vi "Plot V.vi"(7 "Channel number":i32=4, 8 "XY Graph REF":refnum<vi>, 10 "V":bool, 11 "plot setting REF":refnum<vi>) -> ()   [LabVIEW 2023]
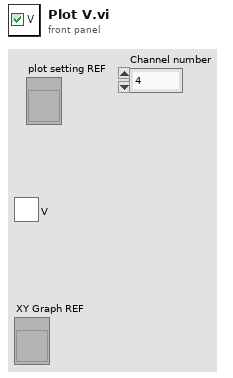
[diagram p1: front panel]
types:
  T1 = cluster{"V plot":bool, "I plot":bool, "Plot colour":u32, "Channel name\n":string}[]
  T2 = cluster{bool, bool, "Plot colour":u32, "Channel name\n":string}
  T3 = cluster{bool, "I plot":bool, "Plot colour":u32, "Channel name\n":string}
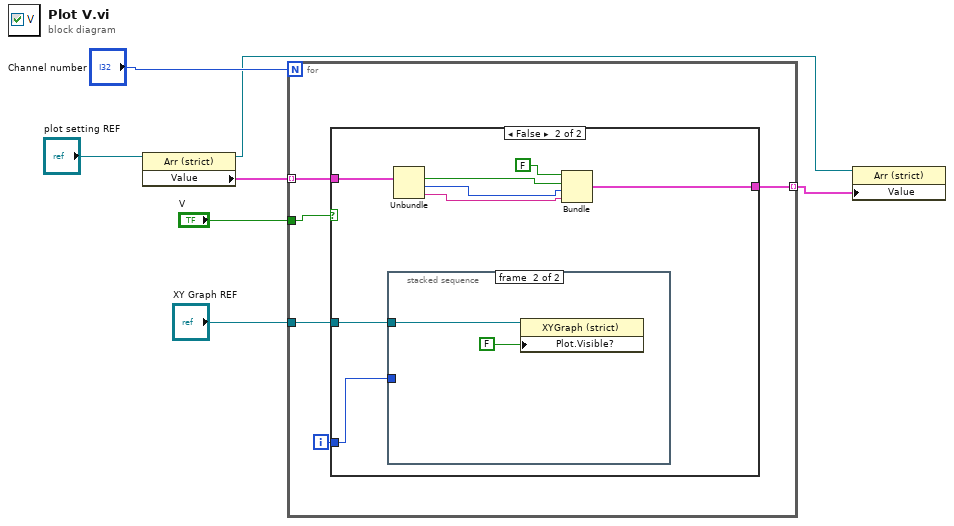
[diagram p0: block diagram]
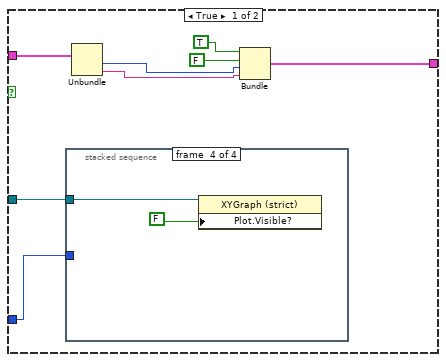
[diagram p2: hidden frame]
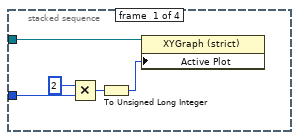
[diagram p3: hidden frame]
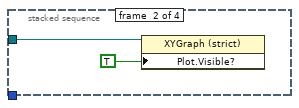
[diagram p4: hidden frame]
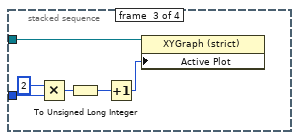
[diagram p5: hidden frame]
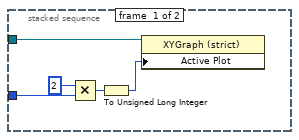
[diagram p6: hidden frame]
diagram:
  n1 = property class="Arr (strict)"(reference="plot setting REF") -> (reference out=w1:refnum<vi>, "Value"=w4:T1)  [unwired: 1 in, 1 out]
  n2 = for {
    N: "Channel number" -> [_]
    tunnel: "XY Graph REF" -> [w9]
    tunnel: w4 -> [w11] mode=indexing
    tunnel: "V" -> [w12]
    tunnel: [w8] -> w2 mode=indexing
    i -> [w10]
    n3 = case shown="False" w12 {
      tunnel: w11 -> [w20 w43]
      tunnel: [w15 w39] -> w8
      tunnel: w10 -> [w13 w37]
      tunnel: w9 -> [w14 w38]
      frame True {
        n4 = stacked-sequence {
          tunnel: w14 -> [w25 w27 w33 w35]
          tunnel: w13 -> [w24 _ w32 _]
          frame #0 {
            n5 = Multiply(x=2, y=w24) -> (x*y=w22:i32)
            n6 = To Unsigned Long Integer(number=w22) -> (unsigned 32bit integer=w21:u32)
            n7 = property class="XYGraph (strict)"(reference=w25, "Active Plot"=w21) -> ()  [unwired: 1 in, 2 out]
          }
          frame #1 {
            n8 = property class="XYGraph (strict)"(reference=w27, "Plot.Visible?"=TRUE ("Plot.Visible")) -> ()  [unwired: 1 in, 2 out]
          }
          frame #2 {
            n9 = Multiply(x=2, y=w32) -> (x*y=w30:i32)
            n10 = To Unsigned Long Integer(number=w30) -> (unsigned 32bit integer=w29:u32)
            n11 = Increment(x=w29) -> (x+1=w28:u32)
            n12 = property class="XYGraph (strict)"(reference=w33, "Active Plot"=w28) -> ()  [unwired: 1 in, 2 out]
          }
          frame #3 {
            n13 = property class="XYGraph (strict)"(reference=w35, "Plot.Visible?"=FALSE ("Plot.Visible")) -> ()  [unwired: 1 in, 2 out]
          }
        }
        n14 = Unbundle(w20) -> ("Plot colour"=w17:u32, "Channel name"=w16:string)  [unwired: 2 out]
        n15 = Bundle(TRUE, FALSE, "Plot colour"=w17, "Channel name"=w16) -> (w15:T2)  [unwired: 1 in]
      }
      frame False {
        n16 = stacked-sequence {
          tunnel: w38 -> [w48 w50]
          tunnel: w37 -> [w47 _]
          frame #0 {
            n17 = Multiply(x=2, y=w47) -> (x*y=w45:i32)
            n18 = To Unsigned Long Integer(number=w45) -> (unsigned 32bit integer=w44:u32)
            n19 = property class="XYGraph (strict)"(reference=w48, "Active Plot"=w44) -> ()  [unwired: 1 in, 2 out]
          }
          frame #1 {
            n20 = property class="XYGraph (strict)"(reference=w50, "Plot.Visible?"=FALSE ("Plot.Visible")) -> ()  [unwired: 1 in, 2 out]
          }
        }
        n21 = Unbundle(w43) -> ("I plot"=w36:bool, "Plot colour"=w41:u32, "Channel name"=w40:string)  [unwired: 1 out]
        n22 = Bundle(FALSE, "I plot"=w36, "Plot colour"=w41, "Channel name"=w40) -> (w39:T3)  [unwired: 1 in]
      }
    }
  }
  n23 = property class="Arr (strict)"(reference=w1, "Value"=w2) -> ()  [unwired: 1 in, 2 out]
